vi "MT Calculate BER After Trigger (User Pattern).vi"(0 "input bit stream":i8[](array[numeric]), 5 "reference bit pattern":i8[](array[numeric]), 7 "BER trigger threshold (0.1)":dbl=0.1 format="%.4f", 9 "confidence (0.95)":dbl=0.95 format="%.4f", 11 "error in (no error)":errorcluster, 13 "reset? (T)":bool=TRUE) -> (4 "BER":dbl=1.0 format="%.4f", 6 "accumulated BER":dbl=1.0 format="%.4f", 8 "trigger found?":bool, 10 "trigger found index (bits)":u32, 15 "error out":errorcluster)   [LabVIEW 2020, in "niDMT.lvlib"]
doc: "This polymorphic instance calculates the average BER against a user-defined sequence. The sequence input in the <B>input bit stream</B> array must be the same as the sequence specified in the <B>reference bit pattern</B> parameter."
uses:
  <vilib>/addons/Modulation/niDMT.lvlib
  <vilib>/addons/Modulation/niAMT.lvlib
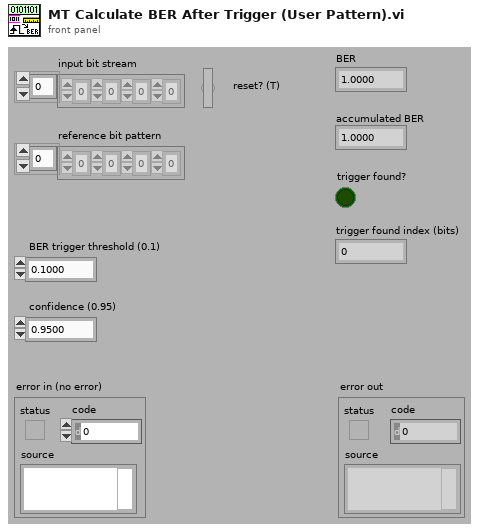
[diagram p1: front panel]
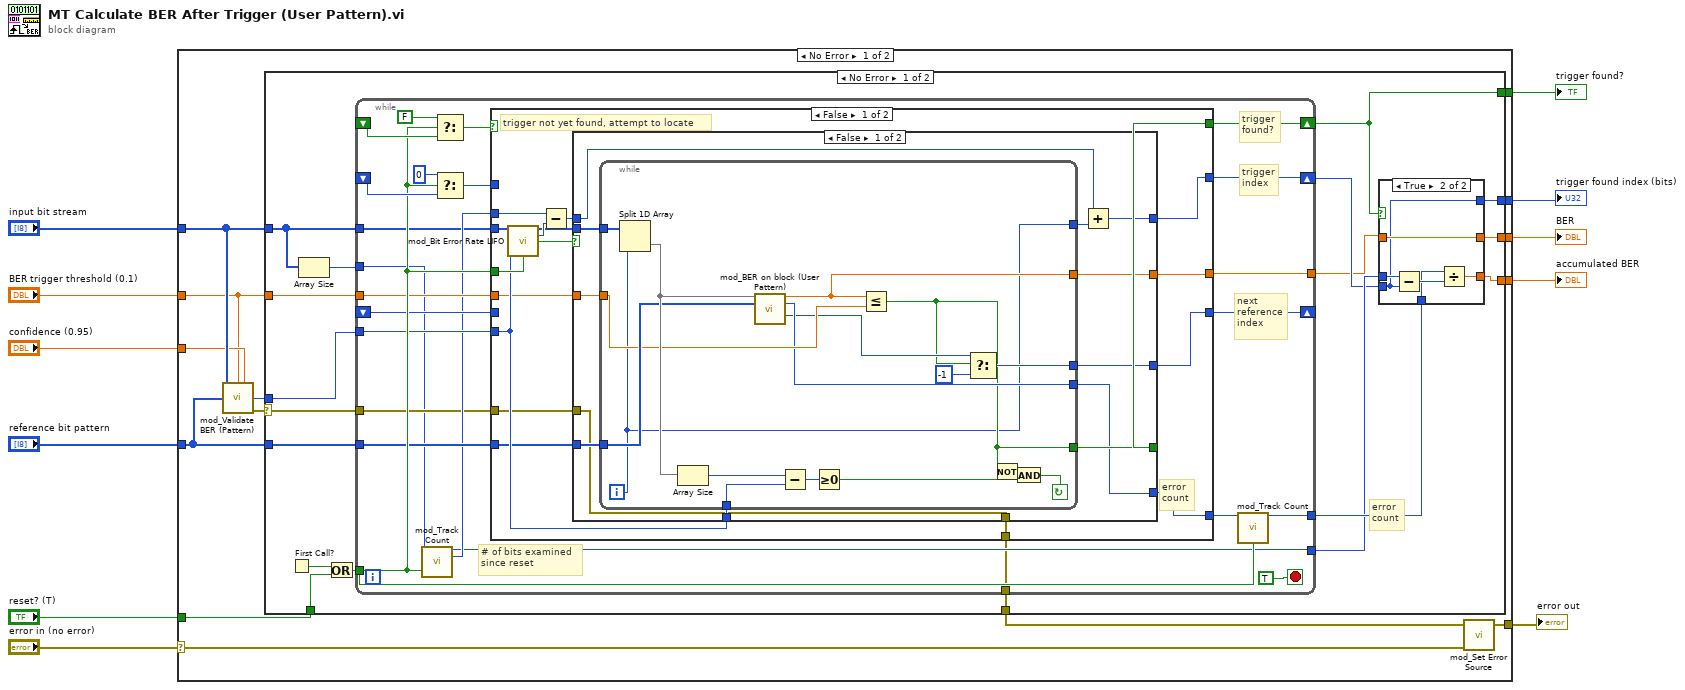
[diagram p0: block diagram]
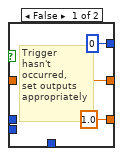
[diagram p2: hidden frame]
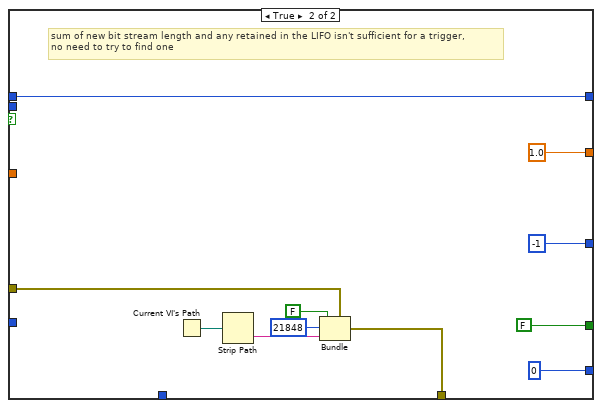
[diagram p3: hidden frame]
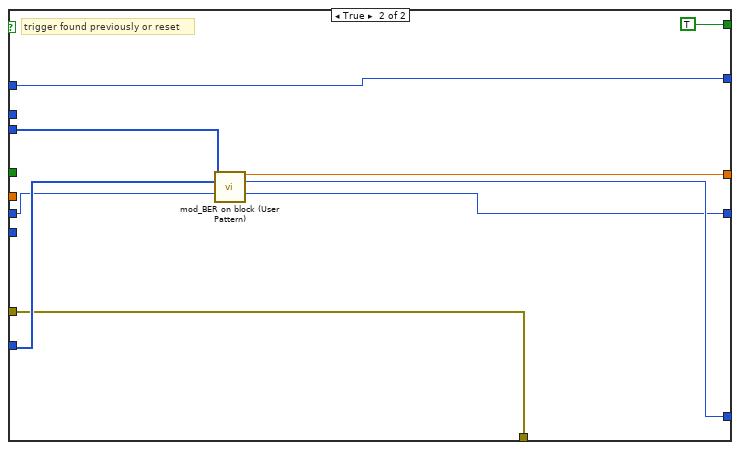
[diagram p4: hidden frame]
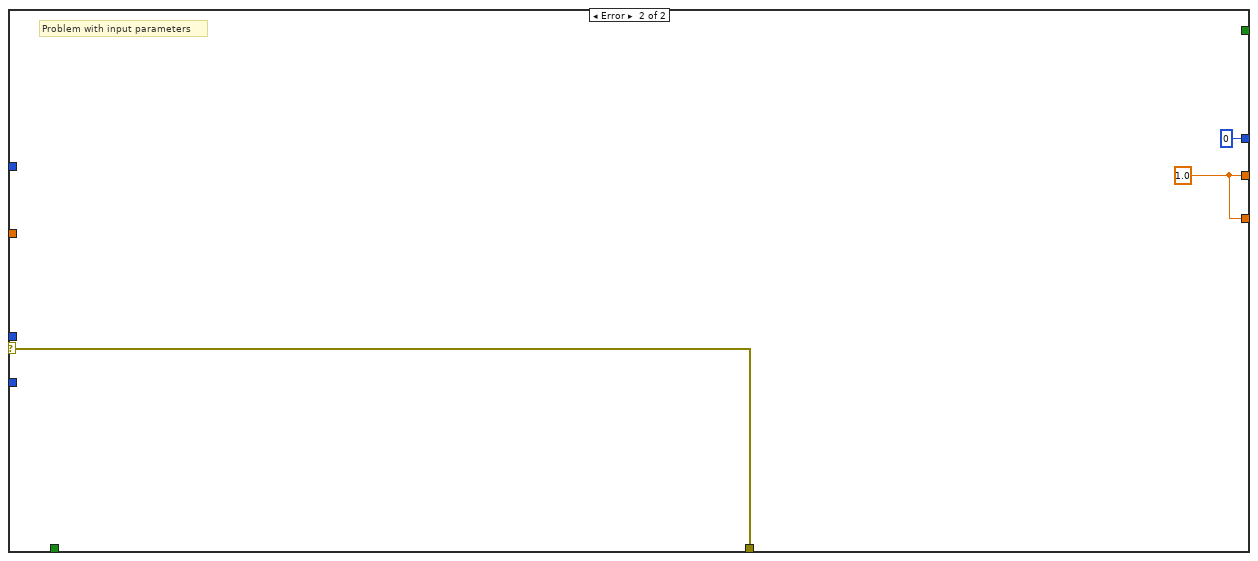
[diagram p5: hidden frame]
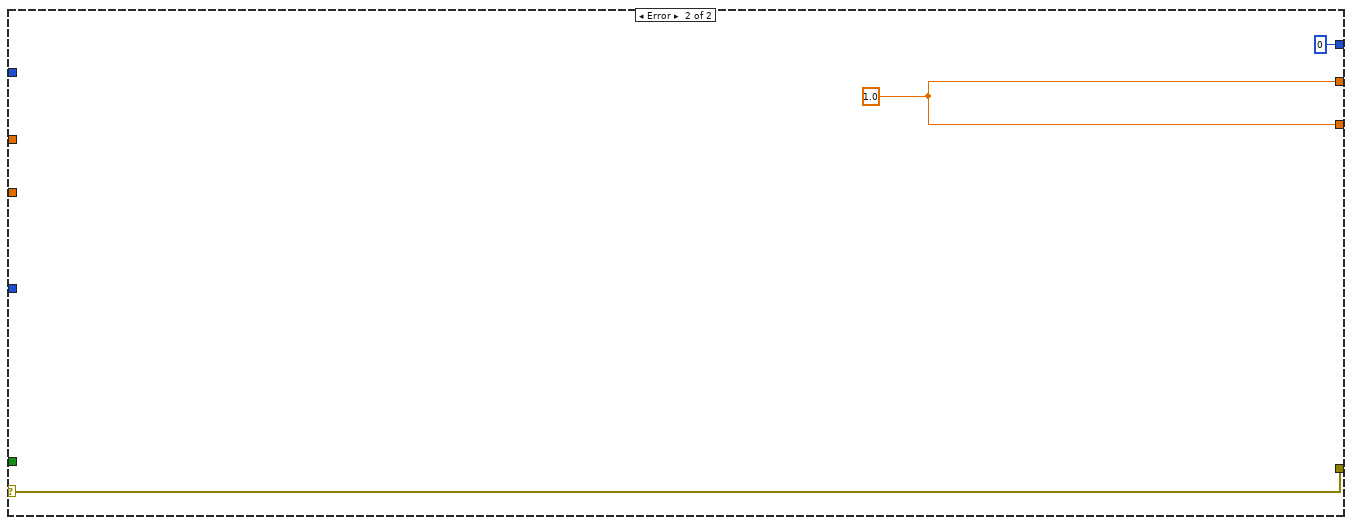
[diagram p6: hidden frame]
diagram:
  n1 = case shown="No Error" "error in (no error)" {
    selector: "error in (no error)" -> [w23 w146]
    tunnel: "reset? (T)" -> [w25 _]
    tunnel: "reference bit pattern" -> [w18 _]
    tunnel: "input bit stream" -> [w19 _]
    tunnel: [w22 w147] -> w8
    tunnel: [w21 w147] -> w7
    tunnel: [w20 w146] -> w5
    tunnel: "BER trigger threshold (0.1)" -> [w13 _]
    tunnel: "confidence (0.95)" -> [w14 _]
    tunnel: [w16 _] -> w1
    tunnel: [w15 u32 0 ("t")] -> w2
    frame No Error {
      n2 = call <vilib>:"mod_Validate BER (Pattern).vi"("Input Bit Stream"=w19, "BER trigger threshold (0.2)"=w13, "confidence (0.95)"=w14, "base user-defined pattern"=w18) -> ("min N"=w12:i32, "error out"=w17:errorcluster)  [unwired: 2 in, 8 out]
      n3 = case shown="No Error" w17 {
        selector: w17 -> [w29 w143]
        tunnel: w25 -> [w43 _]
        tunnel: [w28 w143] -> w24
        tunnel: w18 -> [w31 _]
        tunnel: w19 -> [w27 _]
        tunnel: [w40 w144] -> w22
        tunnel: [w39 w144] -> w21
        tunnel: [w35 _] -> w16
        tunnel: [w41 u32 0 ("t")] -> w15
        tunnel: w13 -> [w33 _]
        tunnel: w12 -> [w30 _]
        frame No Error {
          # "error\ncount"
          n4 = First Call?() -> (First Call?: T/F=w42:bool)
          n5 = Array Size(array=w27) -> (size(s)=w26:i32)
          n6 = Or(x=w42, y=w43) -> (x .or. y?=w34:bool)
          n7 = while {
            tunnel: w34 -> [w65]
            tunnel: w31 -> [w62]
            tunnel: w27 -> [w55]
            shift-right: [w69] -> w35
            shift-left: _ -> [w74]
            tunnel: [w66] -> w38
            tunnel: [w56] -> w37
            shift-right: [w67] -> w36
            shift-left: _ -> [w72]
            tunnel: w30 -> [w63]
            tunnel: w33 -> [w61]
            tunnel: [w60] -> w32
            shift-right: [w59] -> _
            shift-left: _ -> [w58]
            tunnel: w29 -> [w54]
            tunnel: [w53] -> w28
            tunnel: w26 -> [w52]
            stop <- TRUE stop-if-true
            # "# of bits examined \nsince reset"
            # "trigger\nfound?"
            # "trigger\nindex"
            # "next\nreference\nindex"
            n8 = call <vilib>:"mod_Track Count.vi"("Update Count"=w52, "reset? (T)"=w65) -> ("Current Accumulated Count"=w56:u32, "Previously Accumulated"=w57:u32)  [unwired: 12 out]
            n9 = Select(t=FALSE, s=w65, f=w74) -> (s? t:f=w70:bool)
            n10 = Select(t=u32 0, s=w65, f=w72) -> (s? t:f=w68:u32)
            n11 = case shown="False" w70 {
              tunnel: w57 -> [w91 _]
              tunnel: w65 -> [w90 _]
              tunnel: w55 -> [w89 w139]
              tunnel: [w87 TRUE] -> w69
              tunnel: w68 -> [_ w140]
              tunnel: [w84 w140] -> w67
              tunnel: [w86 w136] -> w64
              tunnel: w63 -> [w82 _]
              tunnel: w62 -> [w81 w138]
              tunnel: w61 -> [w80 _]
              tunnel: [w79 w137] -> w60
              tunnel: [w78 w135] -> w59
              tunnel: w58 -> [_ w134]
              tunnel: w54 -> [w77 w133]
              tunnel: [w76 w133] -> w53
              frame False {
                # "error\ncount"
                # "trigger not yet found, attempt to locate"
                n12 = call <vilib>:"mod_Bit Error Rate LIFO.vi"("input bit stream"=w89, "max buffer length"=w82, "reset"=w90) -> ("output bit stream"=w83:i8[], "Old Buffer Length (Prior to New Bits)"=w92:i32, "Updated Buffer Length less \nthan max length"=w88:bool)  [unwired: 10 out]
                n13 = Subtract(x=w91, y=w92) -> (x-y=w85:u32)
                n14 = case shown="False" w88 {
                  tunnel: [w101 FALSE] -> w87
                  tunnel: [w96 u32 0] -> w86
                  tunnel: w85 -> [w103 w130]
                  tunnel: [w104 w130] -> w84
                  tunnel: w83 -> [w102 _]
                  tunnel: w82 -> [w100 _]
                  tunnel: w81 -> [w98 _]
                  tunnel: w80 -> [w97 _]
                  tunnel: [w95 1.0 ("BER")] -> w79
                  tunnel: [w94 -1 ("next reference index")] -> w78
                  tunnel: w77 -> [w93 w123]
                  tunnel: [w93 w122] -> w76
                  frame False {
                    n15 = while {
                      tunnel: w102 -> [w121]
                      tunnel: [w106] -> w101
                      tunnel: w100 -> [w116]
                      tunnel: [w105] -> w99
                      tunnel: w98 -> [w114]
                      tunnel: w97 -> [w113]
                      tunnel: [w111] -> w96
                      tunnel: [w112] -> w95
                      tunnel: [w108] -> w94
                      i -> [w105]
                      stop <- w120 continue-if-true
                      n16 = Split 1D Array(array=w121, index=w105) -> (second subarray=w115:i8[])  [unwired: 1 out]
                      n17 = Array Size(array=w115) -> (size(s)=w118:i32)
                      n18 = call <vilib>:"mod_BER on block (User Pattern).vi"("test bit stream"=w115, "reference bit stream"=w114) -> ("BER"=w112:dbl, "error count (bits)"=w111:u32, "next reference index"=w110:i32)  [unwired: 4 in, 7 out]
                      n19 = Subtract(x=w118, y=w116) -> (x-y=w119:i32)
                      n20 = Greater Or Equal To 0?(x=w119) -> (x >= 0?=w117:bool)
                      n21 = Less Or Equal?(x=w112, y=w113) -> (x <= y?=w106:bool)
                      n22 = Select(t=w110, s=w106, f=-1) -> (s? t:f=w108:i32)
                      n23 = Not(x=w106) -> (.not. x?=w107:bool)
                      n24 = And(x=w107, y=w117) -> (x .and. y?=w120:bool)
                    }
                    n25 = Add(x=w103, y=w99) -> (x+y=w104:u32)
                  }
                  frame True {
                    # "sum of new bit stream length and any retained in the LIFO isn't sufficient for a trigger,\nno need to try to find one"
                    n26 = Current VI's Path() -> (path=w127:path)
                    n27 = Strip Path(path=w127) -> (name=w125:string)  [unwired: 1 out]
                    n28 = Bundle(cluster=w123, "status"=FALSE, "code"=21848, "source"=w125) -> (w122:errorcluster)
                  }
                }
              }
              frame True {
                # "trigger found previously or reset"
                n29 = call <vilib>:"mod_BER on block (User Pattern).vi"("test bit stream"=w139, "reference bit stream"=w138, "start index (reference bit stream)"=w134) -> ("BER"=w137:dbl, "error count (bits)"=w136:u32, "next reference index"=w135:i32)  [unwired: 2 in, 8 out]
              }
            }
            n30 = call <vilib>:"mod_Track Count.vi"("Update Count"=w64, "reset? (T)"=w65) -> ("Current Accumulated Count"=w66:u32)  [unwired: 13 out]
          }
          n31 = case shown="True" w35 {
            tunnel: w37 -> [_ w48]
            tunnel: w38 -> [_ w46]
            tunnel: [w45 w51] -> w39
            tunnel: w36 -> [_ w47]
            tunnel: w32 -> [_ w50]
            tunnel: [w45 w50] -> w40
            tunnel: [u32 0 ("t") w47] -> w41
            frame False {
              w45 = 1.0 ("f")
              # "Trigger\nhasn't \noccurred,\nset outputs\nappropriately"
            }
            frame True {
              n32 = Subtract(x=w48, y=w47) -> (x-y=w49:u32)
              n33 = Divide(x=w46, y=w49) -> (x/y=w51:dbl)
            }
          }
        }
        frame Error {
          w144 = 1.0
          # "Problem with input parameters"
        }
      }
      n34 = call <vilib>:"mod_Set Error Source.vi"("initial error in (no error)"=w23, "final error in (no error)"=w24) -> ("error out"=w20:errorcluster)  [unwired: 3 out]
    }
    frame Error {
      w147 = 1.0
    }
  }
  "error out" <- w5
  "BER" <- w8
  "accumulated BER" <- w7
  "trigger found index (bits)" <- w2
  "trigger found?" <- w1
